vi "Message Handlers.vi"(8 "error in (no error)":errorcluster, 9 "Message Data":variant, 10 "Message":T1, 11 "Network Session Handler in":refnum<class "Network Session Handler.lvclass">) -> (0 "error out":errorcluster, 2 "Number of Active Handlers":i32, 3 "Network Session Handler out":refnum<class "Network Session Handler.lvclass">)   [LabVIEW 2017, in "Network Interface.lvlib" / "Network Session Handler.lvclass"]
uses:
  <vilib>/gpm_packages/@cs/Network-sink/Source/Network Interface/Network Session Handler/Network Session Handler.lvclass
  <vilib>/gpm_packages/@cs/Network-sink/Source/Network Interface/Connection Handler/Message Names ENUM.ctl
  <vilib>/gpm_packages/@cs/Network-sink/Source/Network Interface/Network Session Handler/Network Session Handler.lvclass/Network Session Handler.ctl
  <vilib>/gpm_packages/@cs/Network-sink/Source/Network Interface/Message Queue/Message Queue.lvclass/Message Queue.ctl
  43965cb6-9e37-4e20-8154-84eb15352c07.vi
  <vilib>/gpm_packages/@cs/Network-sink/Source/Network Interface/Message Queue/Protected Enqueue.vi
  <vilib>/gpm_packages/@cs/Network-sink/Source/Network Interface/Connection Handler/Connection Handler.lvclass
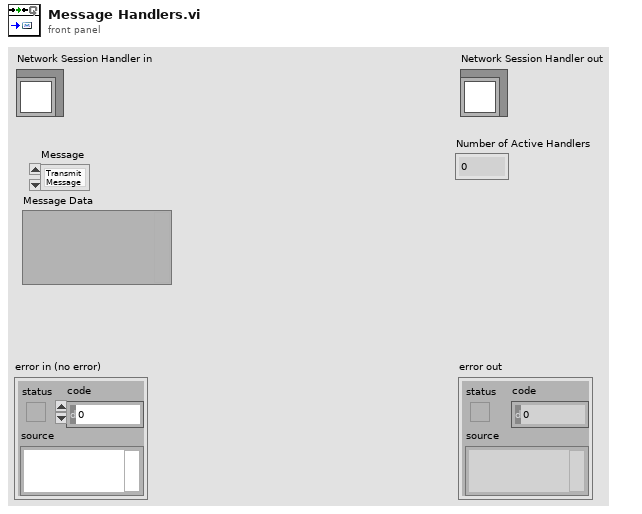
[diagram p1: front panel]
types:
  T1 = typedef "Network Interface.lvlib/Connection Handler.lvclass/Message Names ENUM.ctl" = enum16{"Transmit Message", "Stop"}
  T2 = typedef "Network Interface.lvlib/Network Session Handler.lvclass/Connection Handler.ctl" = cluster{"ID":string, "Handler Queue":refnum<class "Message Queue.lvclass">}
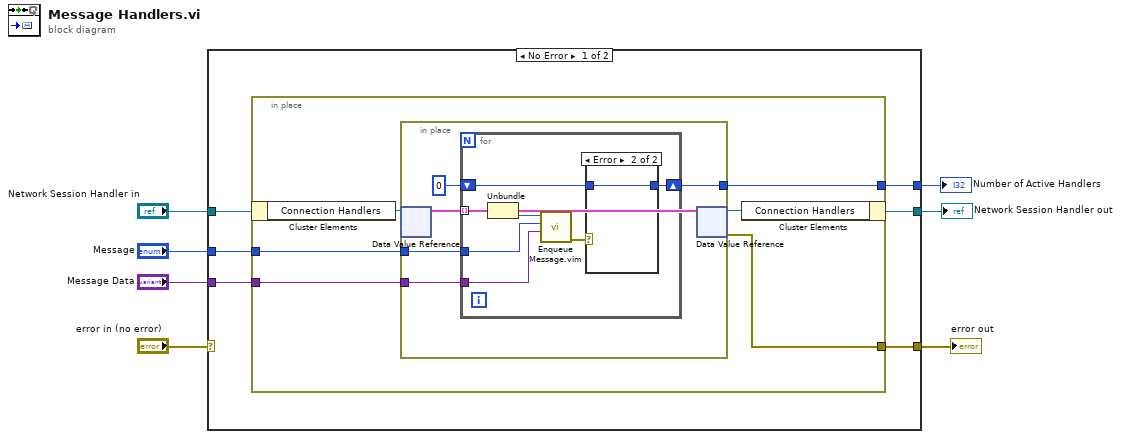
[diagram p0: block diagram]
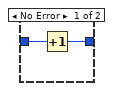
[diagram p2: hidden frame]
diagram:
  n1 = case shown="No Error" "error in (no error)" {
    selector: "error in (no error)" -> [_ w36]
    tunnel: [w9 w36] -> w6
    tunnel: [w10 w35] -> w4
    tunnel: "Network Session Handler in" -> [w13 w35]
    tunnel: "Message" -> [w12 _]
    tunnel: "Message Data" -> [w11 _]
    tunnel: [w8 _] -> w1
    frame No Error {
      n2 = in-place {
        in-place-border: w12 -> [w18]
        in-place-border: w11 -> [w17]
        in-place-border: [w15] -> w9
        in-place-border: [w14] -> w8
        n3 = in-place-cluster #1(w13) -> ("Connection Handlers"=w19:refnum<data-value>)
        n4 = in-place {
          in-place-border: w18 -> [w24]
          in-place-border: w17 -> [w23]
          in-place-border: [w21] -> w14
          n5 = in-place-dvr #2(w19) -> (w20:T2[])  [unwired: 1 out]
          n6 = for {
            tunnel: w20 -> [w28] mode=indexing
            tunnel: w24 -> [w26]
            tunnel: w23 -> [w25]
            shift-right: [w29] -> w21
            shift-left: 0 -> [w30]
            n7 = Unbundle(w28) -> ("Handler Queue"=w27:refnum<class "Message Queue.lvclass">)  [unwired: 1 out]
            n8 = call "Enqueue Message.vim"("Data"=w25, "Msg"=w26, "Message Queue in"=w27) -> ("error out"=w31:errorcluster)  [unwired: 7 in, 1 out]
            n9 = case shown="Error" w31 {
              tunnel: w30 -> [w33 w34]
              tunnel: [w32 w34] -> w29
              frame No Error {
                n10 = Increment(x=w33) -> (x+1=w32:i32)
              }
              frame Error {
              }
            }
          }
          n11 = in-place-dvr #2(w20) -> (w16:refnum<data-value>, w15:errorcluster)
        }
        n12 = in-place-cluster #1("Connection Handlers"=w16) -> (w10:refnum<class "Network Session Handler.lvclass">)
      }
    }
    frame Error {
    }
  }
  "error out" <- w6
  "Network Session Handler out" <- w4
  "Number of Active Handlers" <- w1
